vi "Histogram - Generic.vi"(10 "XYGraph Ref":refnum<vi>, 11 "Matrix":bool[][](array[boolean])) -> (3 "Nb of X per Y":cluster{i32[], i32[]}(graph))   [LabVIEW 2021, in "Bananas.lvlib" / "Pips.lvclass"]
uses:
  Pips.lvclass
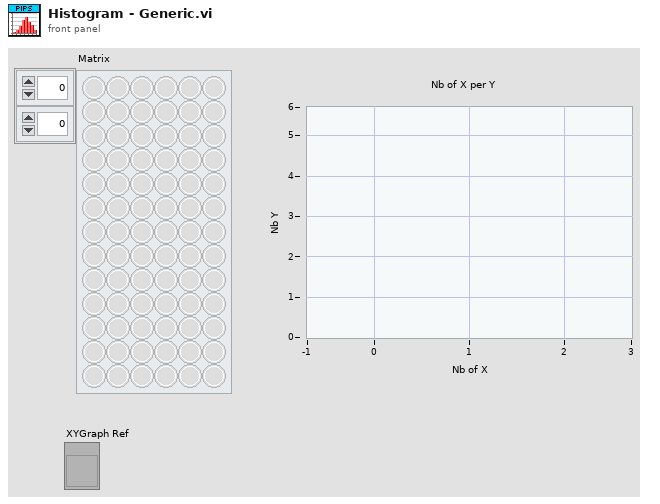
[diagram p1: front panel]
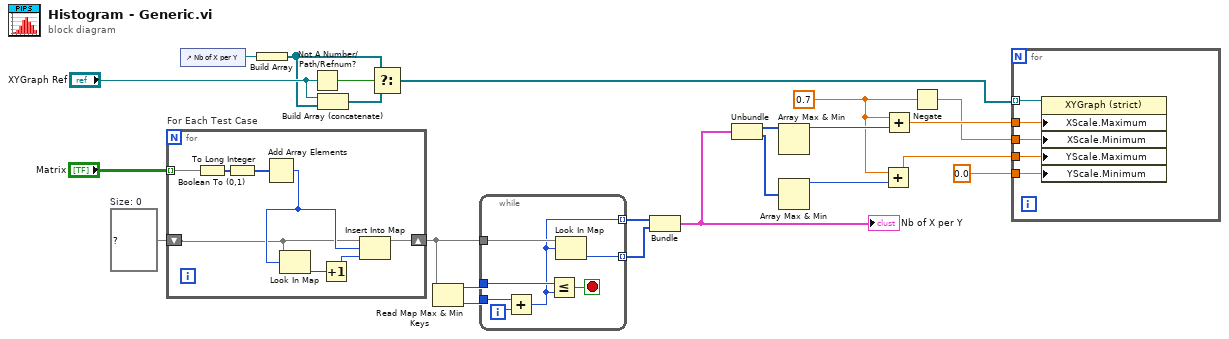
[diagram p0: block diagram]
diagram:
  w3 = map{i32, i32} {}  # Size: 0
  w20 = 0.7 ("Y Scale.Range:Minimum")
  n1 = for "For Each Test Case" {
    tunnel: "Matrix" -> [w29] mode=indexing
    shift-right: [w25] -> w8
    shift-left: w3 -> [w24]
    n2 = Boolean To (0,1)(Boolean=w29) -> (0, 1=w31:i16[])
    n3 = To Long Integer(number=w31) -> (32bit integer=w30:i32[])
    n4 = Add Array Elements(numeric array=w30) -> (sum=w26:i32)
    n5 = Look In Map(map=w24, key=w26) -> (value=w28:i32)  [unwired: 1 in, 1 out]
    n6 = Increment(x=w28) -> (x+1=w27:i32)
    n7 = Insert Into Map(map in=w24, key=w26, value=w27) -> (map out=w25:map{i32, i32})  [unwired: 2 out]
  }
  n8 = control-ref of="Nb of X per Y"() -> (w12:refnum<vi>)
  n9 = Build Array(w12) -> (w11:refnum<vi>[])
  n10 = Not A Number/Path/Refnum?(number/path/refnum="XYGraph Ref") -> (NaN/Path/Refnum?=w16:bool)
  n11 = Build Array (concatenate)("XYGraph Ref", w11) -> (w13:refnum<vi>[])
  n12 = Select(t=w11, s=w16, f=w13) -> (s? t:f=w15:refnum<vi>[])
  n13 = Read Map Max & Min Keys(11:w8) -> (1:w4:i32, 3:w7:i32)
  n14 = while {
    tunnel: w4 -> [w33]
    tunnel: w7 -> [w37]
    tunnel: [w34] -> w6 mode=indexing
    tunnel: w8 -> [w35]
    tunnel: [w32] -> w5 mode=indexing
    i -> [w38]
    stop <- w36 stop-if-true
    n15 = Add(x=w33, y=w38) -> (x+y=w34:i32)
    n16 = Less Or Equal?(x=w37, y=w34) -> (x <= y?=w36:bool)
    n17 = Look In Map(map=w35, key=w34) -> (value=w32:i32)  [unwired: 1 in, 1 out]
  }
  n18 = Bundle(w6, w5) -> (w1:cluster{i32[], i32[]})  [unwired: 1 in]
  "Nb of X per Y" <- w1
  n19 = Unbundle(w1) -> (w10:i32[], w9:i32[])
  n20 = Array Max & Min(array=w10) -> (max value=w22:i32)  [unwired: 3 out]
  n21 = Array Max & Min(array=w9) -> (max value=w19:i32)  [unwired: 3 out]
  n22 = Add(x=w20, y=w19) -> (x+y=w18:dbl)
  n23 = Add(x=w20, y=w22) -> (x+y=w23:dbl)
  n24 = Negate(x=w20) -> (-x=w21:dbl)
  n25 = for {
    tunnel: w23 -> [w43]
    tunnel: w21 -> [w42]
    tunnel: w18 -> [w41]
    tunnel: 0.0 ("Y Scale.Range:Minimum") -> [w40]
    tunnel: w15 -> [w39] mode=indexing
    n26 = property on="Property Node" class="XYGraph (strict)"(reference=w39, "XScale.Maximum"=w43, "XScale.Minimum"=w42, "YScale.Maximum"=w41, "YScale.Minimum"=w40) -> ()  [unwired: 1 in, 2 out]
  }
